vi "Write U8.vi"(8 "error in (no error)":errorcluster, 9 "Numeric":u8, 10 "Tag":string, 11 "Omni_Bus in":refnum<class "Omni_Bus.lvclass">) -> (0 "error out":errorcluster, 3 "Omni_Bus out":refnum<class "Omni_Bus.lvclass">)   [LabVIEW 2021, in "Omni_Bus.lvclass"]
uses:
  Omni_Bus.lvclass
  <vilib>/TSA/Abstract Data Classes/Abs_Types/U8 Integer/Abs_U8 Integer.lvclass
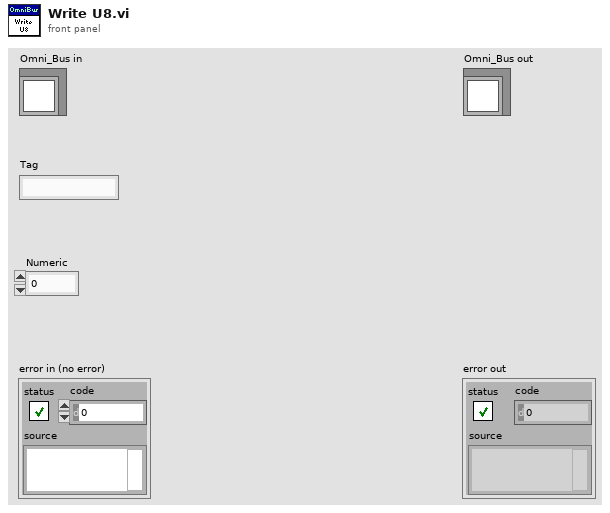
[diagram p1: front panel]
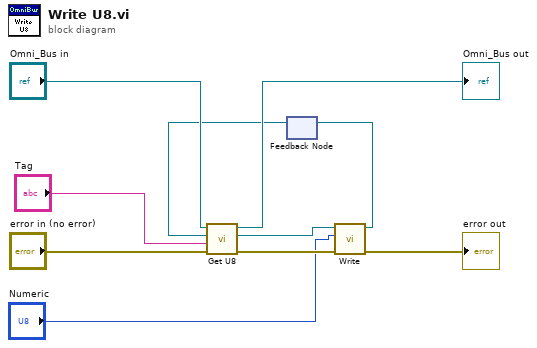
[diagram p0: block diagram]
diagram:
  n1 = feedback #1() -> (w2:refnum<class "Abs_U8 Integer.lvclass">)  [unwired: 1 in]
  n2 = call-dynamic "Get U8.vi"("error in (no error)"="error in (no error)", "Tag"="Tag", "Value Type"=w2, "Var Bus in"="Omni_Bus in") -> ("error out"=w6:errorcluster, "Value Out"=w3:refnum<class "Abs_U8 Integer.lvclass">, "Var Bus out"=→"Omni_Bus out":refnum<class "Omni_Bus.lvclass">)  [unwired: 5 in]
  n3 = call-dynamic "Write.vi"("error in (no error)"=w6, "Value"="Numeric", "Double Float.lvclass_340760 in"=w3) -> ("error out"=→"error out":errorcluster, "Double Float.lvclass_340760 out"=w4:refnum<class "Abs_U8 Integer.lvclass">)  [unwired: 7 in]
  n4 = feedback-in #1(w4) -> ()
